vi "Tester.vi"() -> ()   [LabVIEW 2024, in "AddNewModule.lvlib"]
uses:
  AddNewModule.lvlib
panel:
  out "error out":errorcluster
  in  "ModuleParams":T1={"Template Class Path"=path "C:/Github/JQMH/Scripting/templates/TemplateModule/TemplateModule.lvclass", "Tester Path"=path "C:/Github/JQMH/Scripting/templates/TemplateModule/Tester_TemplatModule.vi", "Name"="James"}
  in  "Save Folder":path=path "C:/Github/JQMH/Scripting/Module/Testing/James"
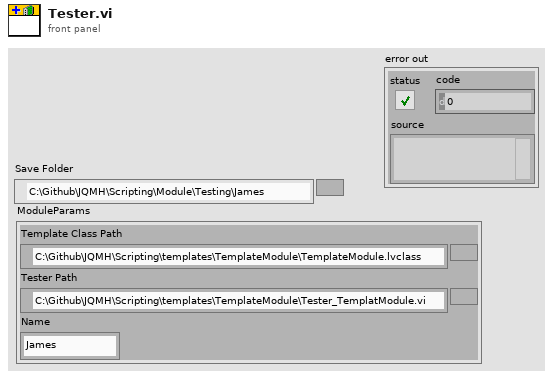
[diagram p1: front panel]
types:
  T1 = cluster{"Template Class Path":path, "Tester Path":path, "Name":string}
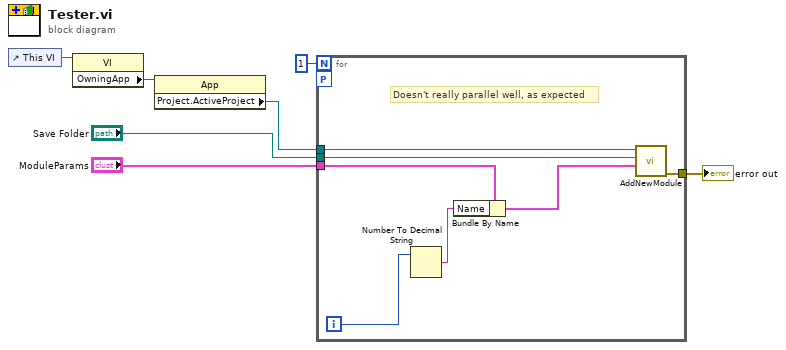
[diagram p0: block diagram]
diagram:
  n1 = control-ref of="This VI"() -> (w6:refnum<vi>)
  n2 = property class="VI"(reference=w6) -> ("OwningApp"=w5:refnum<vi>)  [unwired: 1 in, 2 out]
  n3 = property class="App"(reference=w5) -> ("Project.ActiveProject"=w4:refnum<vi>)  [unwired: 1 in, 2 out]
  n4 = for {
    N: 1 -> [_]
    tunnel: "Save Folder" -> [w14]
    tunnel: w4 -> [w13]
    tunnel: [w12] -> w3
    tunnel: "ModuleParams" -> [w11]
    workers-P: _ -> [_]
    i -> [w8]
    # "Doesn't really parallel well, as expected"
    n5 = Number To Decimal String(number=w8) -> (decimal integer string=w9:string)  [unwired: 1 in]
    n6 = Bundle By Name(cluster=w11, "Name"=w9) -> (w10:T1)
    n7 = call "AddNewModule.vi"("ModuleParams"=w10, "Save Folder"=w14, "Project in"=w13) -> ("error out"=w12:errorcluster)  [unwired: 7 in, 1 out]
  }
  "error out" <- w3
